vi "unpack autonomous file.vi"(11 "file path in":path) -> (3 "command/parameter array out":string[][](array[string]))   [LabVIEW 2011]
uses:
  <vilib>/Utility/file.llb/Read From Spreadsheet File (string).vi
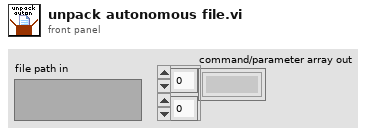
[diagram p1: front panel]
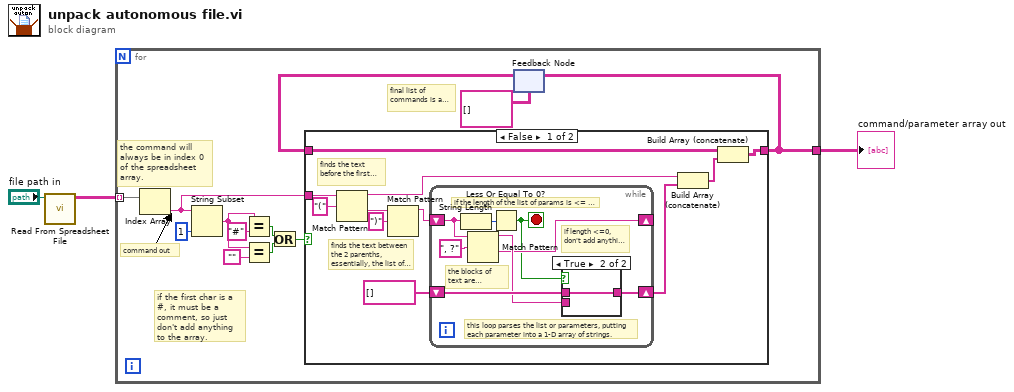
[diagram p0: block diagram]
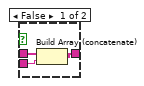
[diagram p2: hidden frame]
diagram:
  n1 = call-poly <vilib>:"Read From Spreadsheet File.vi"("file path (dialog if empty)"="file path in") -> ("all rows"=w2:string[][])  [unwired: 6 in, 4 out]
  n2 = for {
    tunnel: w2 -> [w15] mode=indexing
    tunnel: [w9] -> w3
    # "final list of commands is a 2-D array of strings."
    # "if the first char is a #, it must be a comment, so just don't add anything to the array."
    # "command out"
    # "the command will always be in index 0 of the spreadsheet array."
    n3 = Index Array(array=w15) -> (element=w12:string)  [unwired: 1 in]
    n4 = String Subset(string=w12, length (rest)=1 ("length (rest)")) -> (substring=w7:string)  [unwired: 1 in]
    n5 = Equal?(x=w7, y="#") -> (x = y?=w6:bool)
    n6 = Equal?(x=w7, y="") -> (x = y?=w5:bool)
    n7 = Or(x=w6, y=w5) -> (x .or. y?=w4:bool)
    n8 = feedback #1(string[][] []) -> (w10:string[][])
    n9 = case shown="False" w4 {
      tunnel: w12 -> [w26 _]
      tunnel: w10 -> [w17 w39]
      tunnel: [w16 w39] -> w9
      frame False {
        # "finds the text between the 2 parenths, essentially, the list of parameters"
        # "finds the text before the first parenth, the function name"
        n10 = Match Pattern(string=w26, regular expression="(") -> (before substring=w19:string, after substring=w24:string)  [unwired: 1 in, 2 out]
        n11 = Match Pattern(string=w24, regular expression=")") -> (before substring=w21:string)  [unwired: 1 in, 3 out]
        n12 = while {
          shift-right: [w29] -> _
          shift-left: w21 -> [w33]
          shift-right: [w27] -> w20
          shift-left: string[] [] -> [w31]
          stop <- w28 stop-if-true
          # "if length <=0, don't add anything to the array of parameters."
          # "this loop parses the list or parameters, putting each parameter into a 1-D array of strings."
          # "the blocks of text are seperated by ,[space] or ,."
          # "if the length of the list of params is <= 0, stop."
          n13 = String Length(string=w33) -> (length=w34:i32)
          n14 = Match Pattern(string=w33, regular expression=", ?") -> (before substring=w30:string, after substring=w29:string)  [unwired: 1 in, 2 out]
          n15 = Less Or Equal To 0?(x=w34) -> (x <= 0?=w28:bool)
          n16 = case shown="True" w28 {
            tunnel: w31 -> [w36 w38]
            tunnel: w30 -> [w37 _]
            tunnel: [w35 w38] -> w27
            frame False {
              n17 = Build Array (concatenate)(w36, w37) -> (w35:string[])
            }
            frame True {
            }
          }
        }
        n18 = Build Array (concatenate)(w19, w20) -> (w18:string[])
        n19 = Build Array (concatenate)(w17, w18) -> (w16:string[][])
      }
      frame True {
        # "First character of the line was a '#', so don't do anything"
      }
    }
    n20 = feedback-in #1(w9) -> ()
  }
  "command/parameter array out" <- w3
